vi "报文获取.vi"(0 "MainPage":refnum<class "MainPage.lvclass"> caption="类") -> (9 "寄存器模拟":u16[](array[numeric]), 11 "状态信息":T1, 14 "流水显示":string, 16 "未知记录":T2(array[cluster]), 17 "03记录":T2(array[cluster]), 18 "06记录":T2(array[cluster]), 19 "16记录":T2(array[cluster]))   [LabVIEW 2019, in "MainPage.lvlib" / "MainPage.lvclass"]
uses:
  MainPage.lvclass
  714c8231-3ad1-446b-bf86-c268c1036eb9.vi
  <vilib>/regexp/Match Regular Expression.xnode
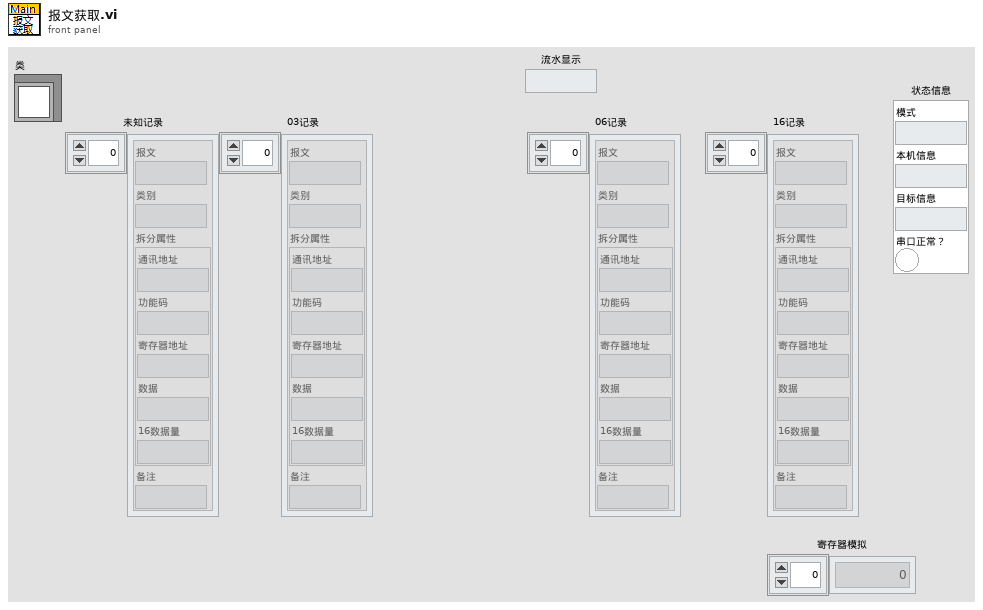
[diagram p1: front panel]
types:
  T1 = cluster{"模式":string, "本机信息":string, "目标信息":string, "串口正常？":bool}
  T2 = cluster{"报文":string, "类别":string, "拆分属性":cluster{"通讯地址":string, "功能码":string, "寄存器地址":string, "数据":string, "16数据量":string}, "备注":string}[]
  T3 = typedef "MainPage.lvlib/MainPage.lvclass/DataRef_通讯接口.ctl" = cluster{"连接方式":enum16{"网口(客服端)", "网口(服务端)", "串口"}, "VISA串口名称":refnum<visa-resource-name>, "服务端识别":cluster{"本机IP":string, "本机端口":u16, "当前目标":string}, "客服端识别":cluster{"客P-主IP:Port":string}, "服务端记录":cluster{"服务端侦听ID":refnum<k5>, "服务端接口记录":map{string, cluster{"连接ID":refnum<k5>}}}, "客服端记录":map{string, cluster{"连接ID":refnum<k5>}}}
  T4 = typedef "MainPage.lvlib/MainPage.lvclass/DataRef_通讯接口数据记录.ctl" = cluster{"串口反馈":cluster{"串口正常？":bool, "寄存器模拟":u16[], "报文信息记录":string[][]}, "服务端记录":map{string, cluster{"寄存器模拟":u16[], "串口正常？":bool, "报文信息记录":string[][]}}, "客服端记录":map{string, cluster{"寄存器模拟":u16[], "串口正常？":bool, "报文信息记录":string[][]}}}
  T5 = map{string, cluster{"寄存器模拟":u16[], "串口正常？":bool, "报文信息记录":string[][]}}
  T6 = cluster{"寄存器模拟":u16[], "串口正常？":bool, "报文信息记录":string[][]}
  T7 = cluster{"报文":string, "类别":string, "拆分属性":cluster{"通讯地址":string, "功能码":string, "寄存器地址":string, "数据":string, "16数据量":string}, "备注":string}
  T8 = cluster{string, "Intf Inst Name":string, string, "串口正常？":bool}
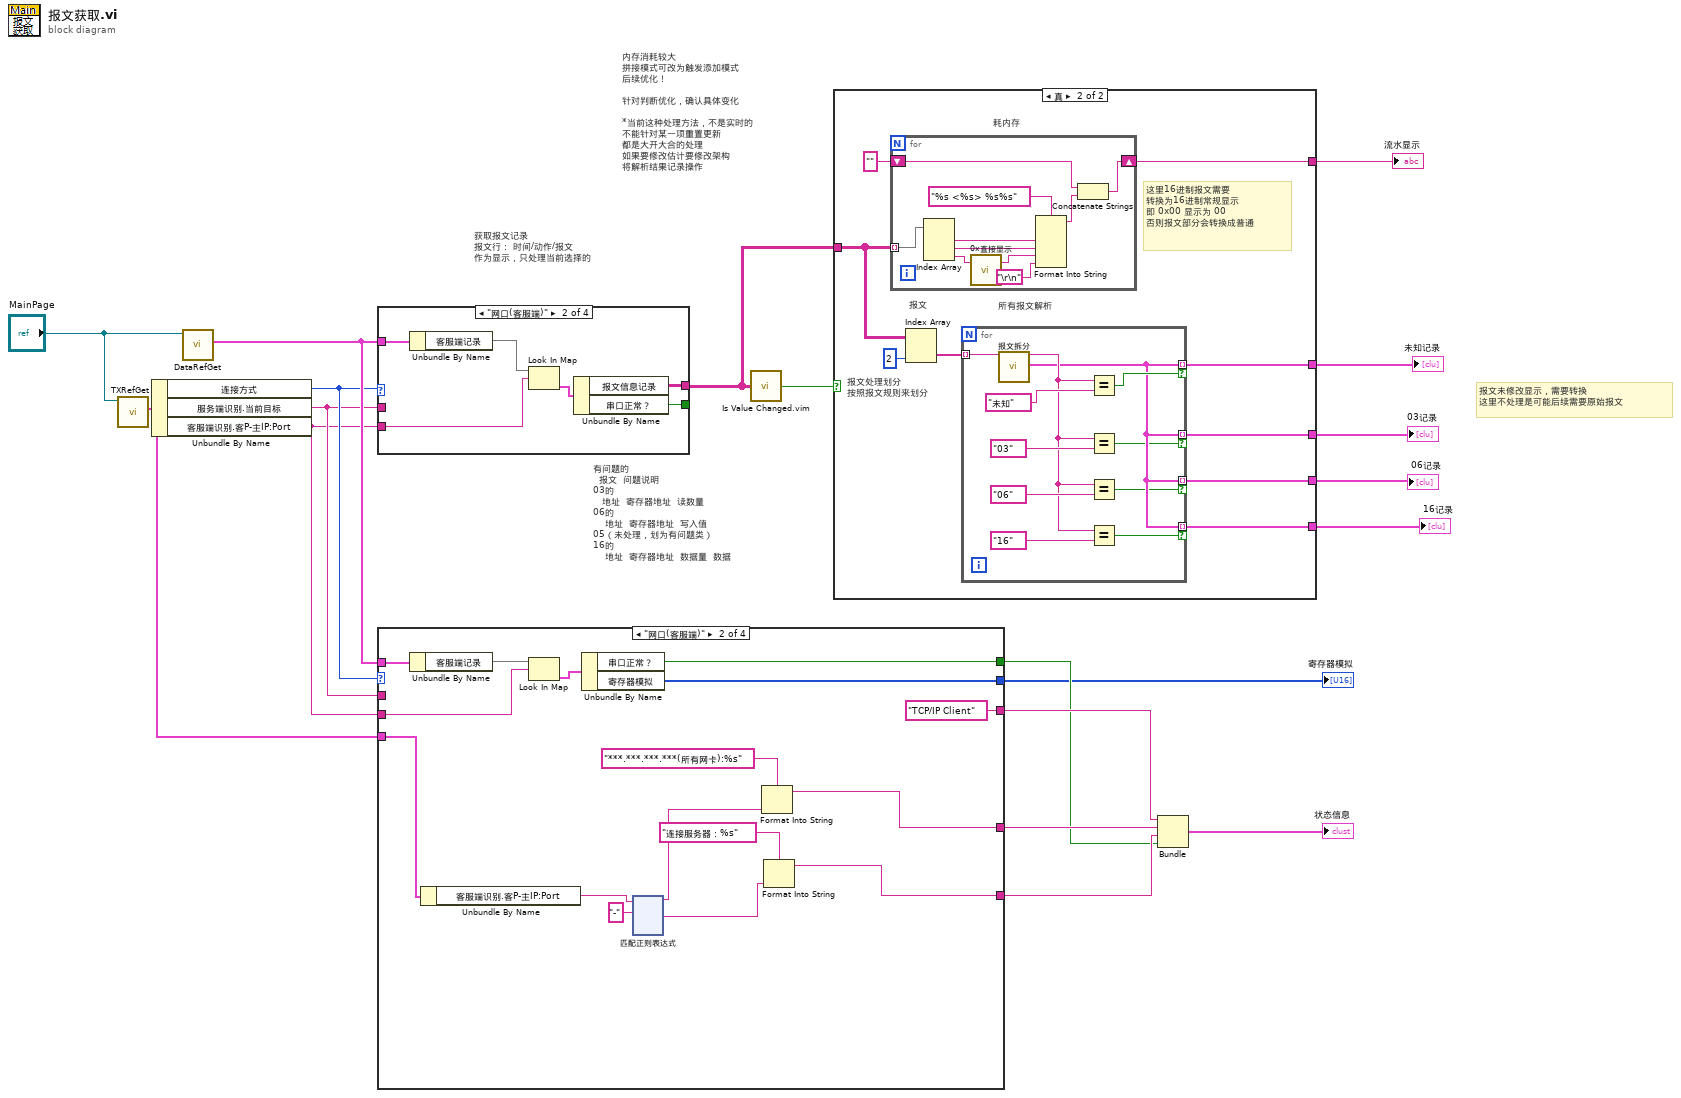
[diagram p0: block diagram]
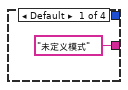
[diagram p2: hidden frame]
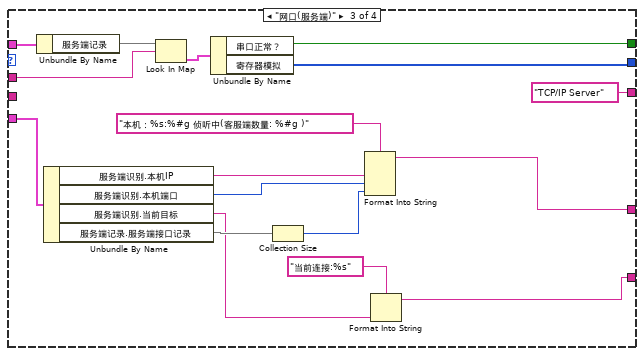
[diagram p3: hidden frame]
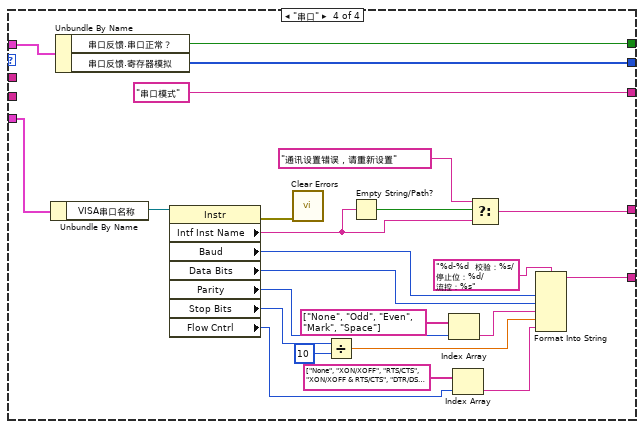
[diagram p4: hidden frame]
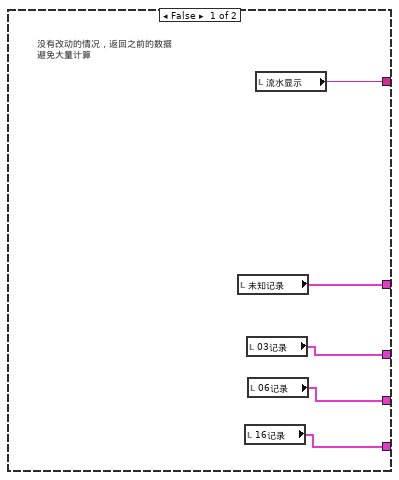
[diagram p5: hidden frame]
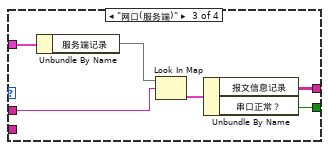
[diagram p7: hidden frame]
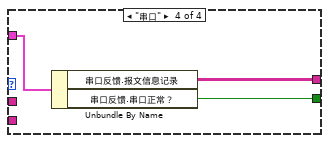
[diagram p8: hidden frame]
diagram:
  # "报文未修改显示，需要转换\n这里不处理是可能后续需要原始报文"
  # "有问题的\n  报文  问题说明\n03的\n   地址  寄存器地址  读数量\n06的\n    地址  寄存器地址  写入值\n05（未处理，划为有问题类）\n16的\n    地址  寄存器地址  数据量  数据"
  # "内存消耗较大\n拼接模式可改为触发添加模式\n后续优化！\n\n针对判断优化，确认具体变化\n\n*当前这种处理方法，不是实时的\n不能针对某一项重置更新\n都是大开大合的处理\n如果要修改估计要修改架构\n将解析结果记录操作"
  # "获取报文记录\n报文行： 时间/动作/报文\n作为显示，只处理当前选择的"
  n1 = call-dynamic "TXRefGet.vi"("MainPage 输入"="MainPage") -> ("通讯接口数据"=w7:T3)  [unwired: 6 in, 4 out]
  n2 = Unbundle By Name(w7) -> ("连接方式"=w10:enum16{"网口(客服端)", "网口(服务端)", "串口"}, "服务端识别.当前目标"=w9:string, "客服端识别.客P-主IP:Port"=w8:string)
  n3 = call-dynamic "DataRefGet.vi"("MainPage 输入"="MainPage") -> ("通讯接口记录"=w11:T4)  [unwired: 6 in, 4 out]
  n4 = case shown="\"网口(客服端)\"" w10 {
    tunnel: w11 -> [_ w25 w29 w34]
    tunnel: w8 -> [_ w23 _ _]
    tunnel: [_ w21 w28 w33] -> w17
    tunnel: w9 -> [_ _ w27 _]
    tunnel: [_ w20 w26 w32] -> _
    frame Default {
    }
    frame "网口(客服端)" {
      n5 = Unbundle By Name(w25) -> ("客服端记录"=w24:T5)
      n6 = Look In Map(map=w24, key=w23) -> (value=w22:T6)  [unwired: 1 in, 1 out]
      n7 = Unbundle By Name(w22) -> ("报文信息记录"=w21:string[][], "串口正常？"=w20:bool)
    }
    frame "网口(服务端)" {
      n8 = Unbundle By Name(w29) -> ("服务端记录"=w31:T5)
      n9 = Look In Map(map=w31, key=w27) -> (value=w30:T6)  [unwired: 1 in, 1 out]
      n10 = Unbundle By Name(w30) -> ("报文信息记录"=w28:string[][], "串口正常？"=w26:bool)
    }
    frame "串口" {
      n11 = Unbundle By Name(w34) -> ("串口反馈.报文信息记录"=w33:string[][], "串口反馈.串口正常？"=w32:bool)
    }
  }
  n12 = case shown="\"网口(客服端)\"" w10 {
    tunnel: w11 -> [_ w51 w180 w206]
    tunnel: w8 -> [_ w49 _ _]
    tunnel: w9 -> [_ _ w179 _]
    tunnel: [_ w47 w178 w205] -> w3
    tunnel: w7 -> [_ w45 w176 w186]
    tunnel: ["未定义模式" "TCP/IP Client" "TCP/IP Server" "串口模式"] -> w6
    tunnel: [_ w43 w172 w185] -> w5
    tunnel: [_ w41 w167 w184] -> w4
    tunnel: [_ w40 w166 w183] -> w1
    frame Default {
    }
    frame "网口(客服端)" {
      n13 = Unbundle By Name(w51) -> ("客服端记录"=w50:T5)
      n14 = Unbundle By Name(w45) -> ("客服端识别.客P-主IP:Port"=w39:string)
      n15 = Look In Map(map=w50, key=w49) -> (value=w48:T6)  [unwired: 1 in, 1 out]
      n16 = Unbundle By Name(w48) -> ("串口正常？"=w47:bool, "寄存器模拟"=w40:u16[])
      n17 = xnode "匹配正则表达式"("输入字符串"=w39, "正则表达式"="-") -> ("匹配之前"=w37:string, "匹配之后"=w36:string)  [unwired: 4 in, 3 out]
      n18 = Format Into String(format string="***.***.***.***(所有网卡):%s" ("格式字符串"), w37) -> (resulting string=w43:string)  [unwired: 2 in, 1 out]
      n19 = Format Into String(format string="连接服务器：%s" ("格式字符串"), w36) -> (resulting string=w41:string)  [unwired: 2 in, 1 out]
    }
    frame "网口(服务端)" {
      n20 = Unbundle By Name(w180) -> ("服务端记录"=w182:T5)
      n21 = Unbundle By Name(w176) -> ("服务端识别.本机IP"=w175:string, "服务端识别.本机端口"=w174:u16, "服务端识别.当前目标"=w168:string, "服务端记录.服务端接口记录"=w171:map{string, cluster{"连接ID":refnum<k5>}})
      n22 = Look In Map(map=w182, key=w179) -> (value=w181:T6)  [unwired: 1 in, 1 out]
      n23 = Unbundle By Name(w181) -> ("串口正常？"=w178:bool, "寄存器模拟"=w166:u16[])
      n24 = Collection Size(1:w171) -> (0:w170:i32)
      n25 = Format Into String(format string="本机：%s:%#g 侦听中(客服端数量: %#g )" ("格式字符串"), w175, w174, w170) -> (resulting string=w172:string)  [unwired: 2 in, 1 out]
      n26 = Format Into String(format string="当前连接:%s" ("格式字符串"), w168) -> (resulting string=w167:string)  [unwired: 2 in, 1 out]
    }
    frame "串口" {
      n27 = Unbundle By Name(w186) -> ("VISA串口名称"=w192:refnum<visa-resource-name>)
      n28 = Unbundle By Name(w206) -> ("串口反馈.串口正常？"=w205:bool, "串口反馈.寄存器模拟"=w183:u16[])
      n29 = property class="Instr"(reference=w192) -> (error out=w201:errorcluster, "Intf Inst Name"=w203:string, "Baud"=w193:u32, "Data Bits"=w194:u16, "Parity"=w196:u16, "Stop Bits"=w199:u16, "Flow Cntrl"=w197:u16)  [unwired: 1 in, 1 out]
      n30 = call <vilib>:"Clear Errors.vi"("error in (no error)"=w201) -> ()  [unwired: 5 in, 2 out]
      n31 = Divide(x=w199, y=u16 10) -> (x/y=w200:dbl)
      n32 = Empty String/Path?(string/path=w203) -> (empty?=w202:bool)
      n33 = Index Array(array=string[] ["None", "Odd", "Even", "Mark", "Space"] ("校验"), index=w196) -> (element=w195:string)
      n34 = Index Array(array=string[] ["None", "XON/XOFF", "RTS/CTS", "XON/XOFF & RTS/CTS", "DTR/DSR", "XON/XOFF & DTR/DSR"] ("流控"), index=w197) -> (element=w198:string)
      n35 = Select(t="通讯设置错误，请重新设置", s=w202, f=w203) -> (s? t:f=w185:string)
      n36 = Format Into String(format string="%d-%d  校验：%s/停止位：%d/流控：%s" ("格式字符串"), w193, w194, w195, w200, w198) -> (resulting string=w184:string)  [unwired: 2 in, 1 out]
    }
  }
  "寄存器模拟" <- w1
  n37 = call "Is Value Changed.vim"("value"=w17) -> ("changed or first call?"=w18:bool)
  n38 = case shown="真" w18 {
    tunnel: w17 -> [_ w218]
    tunnel: [w211 w219] -> w16
    tunnel: [w210 w215] -> w15
    tunnel: [w209 w214] -> w12
    tunnel: [w208 w213] -> w13
    tunnel: [w207 w212] -> w14
    frame False {
      # "没有改动的情况，返回之前的数据\n避免大量计算"
      n39 = local read "未知记录"() -> (w210:T2)
      n40 = local read "16记录"() -> (w209:T2)
      n41 = local read "03记录"() -> (w207:T2)
      n42 = local read "06记录"() -> (w208:T2)
      n43 = local read "流水显示"() -> (w211:string)
    }
    frame True {
      # "所有报文解析"
      # "这里16进制报文需要\n转换为16进制常规显示\n即 0x00 显示为 00\n否则报文部分会转换成普通"
      # "报文处理划分\n按照报文规则来划分"
      # "报文"
      # "耗内存"
      n44 = for {
        tunnel: w218 -> [w241] mode=indexing
        shift-right: [w235] -> w219
        shift-left: "" -> [w234]
        n45 = Index Array(array=w241) -> (element #1=w240:string, element #2=w239:string, element #3=w233:string)  [unwired: 3 in]
        n46 = call "0x直接显示.vi"("普通字符串"=w233) -> ("0x普通字符串"=w232:string)  [unwired: 18 in]
        n47 = Format Into String(format string="%s <%s> %s%s" ("格式字符串"), w240, w239, w232, "\r\n") -> (resulting string=w236:string)  [unwired: 2 in, 1 out]
        n48 = Concatenate Strings(w234, w236) -> (w235:string)
      }
      n49 = Index Array(array=w218, index (col)=2 ("禁用的索引 (列)")) -> (element=w216:string[])  [unwired: 1 in]
      n50 = for {
        tunnel: w216 -> [w231] mode=indexing
        tunnel: [w224] -> w215 mode=indexing if=w229
        tunnel: [w224] -> w212 mode=indexing if=w222
        tunnel: [w224] -> w213 mode=indexing if=w223
        tunnel: [w224] -> w214 mode=indexing if=w221
        n51 = call "报文拆分.vi"("报文"=w231) -> ("类别"=w225:string, "拆分报告"=w224:T7)  [unwired: 17 in]
        n52 = Equal?(x=w225, y="未知" ("类别")) -> (x = y?=w229:bool)
        n53 = Equal?(x=w225, y="03" ("类别")) -> (x = y?=w222:bool)
        n54 = Equal?(x=w225, y="06" ("类别")) -> (x = y?=w223:bool)
        n55 = Equal?(x=w225, y="16" ("类别")) -> (x = y?=w221:bool)
      }
    }
  }
  "流水显示" <- w16
  "未知记录" <- w15
  "03记录" <- w14
  "06记录" <- w13
  "16记录" <- w12
  n56 = Bundle(w6, "Intf Inst Name"=w5, w4, "串口正常？"=w3) -> (→"状态信息":T8)  [unwired: 1 in]
